vi "Generate Data.vi"(8 "error in (no error)":errorcluster, 11 "String Data in":refnum<class "String Data.lvclass">) -> (0 "error out":errorcluster, 3 "String Data out":refnum<class "String Data.lvclass">)   [LabVIEW 2023, in "String Data.lvclass"]
uses:
  String Data.lvclass
  String Data.lvclass/String Data.ctl
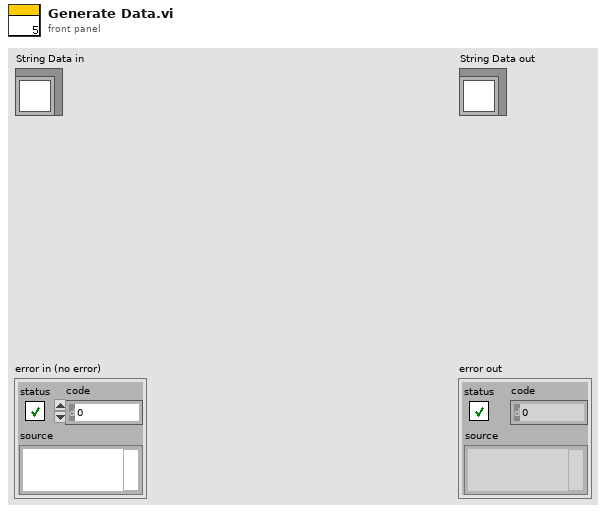
[diagram p1: front panel]
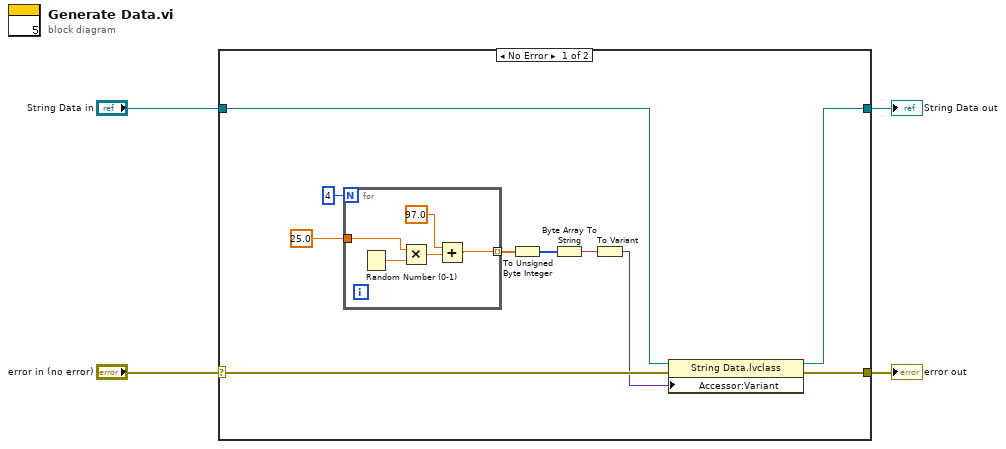
[diagram p0: block diagram]
diagram:
  n1 = case shown="No Error" "error in (no error)" {
    selector: "error in (no error)" -> [w14 w21]
    tunnel: [w8 w21] -> w3
    tunnel: [w5 w20] -> w1
    tunnel: "String Data in" -> [w7 w20]
    frame No Error {
      n2 = for {
        N: 4 -> [_]
        tunnel: 25.0 -> [w18]
        tunnel: [w15] -> w11 mode=indexing
        n3 = Random Number (0-1)() -> (number: 0 to 1=w19:dbl)
        n4 = Multiply(x=w18, y=w19) -> (x*y=w17:dbl)
        n5 = Add(x=97.0, y=w17) -> (x+y=w15:dbl)
      }
      n6 = To Unsigned Byte Integer(number=w11) -> (unsigned 8bit integer=w10:u8[])
      n7 = Byte Array To String(unsigned byte array=w10) -> (string=w9:string)
      n8 = To Variant(anything=w9) -> (Variant=w6:variant)
      n9 = property class="String Data.lvclass"(reference=w7, error in=w14, "Accessor:Variant"=w6) -> (reference out=w5:refnum<class "String Data.lvclass">, error out=w8:errorcluster)
    }
    frame Error {
    }
  }
  "error out" <- w3
  "String Data out" <- w1
